vi "CALC_TRAN_TIME_SPAN_QUES.vi"(0 "VISA IN":refnum<visa-resource-name>, 5 "error in":errorcluster, 7 "Channel":i32) -> (11 "min":dbl, 13 "max":dbl, 14 "VISA Out":refnum<visa-resource-name>, 19 "error out":errorcluster)   [LabVIEW 2018, in "PNA-X.lvlib"]
doc: "CALCulate<cnum>:TRANsform:TIME:SPAN <num> \n1570\n\n(Read-Write) Sets the span time for time domain measurements. \nSee Critical Note \nParameters \n<cnum> Channel number of the measurement. There must be a selected measurement \non that channel. If unspecified, <cnum> is set to 1. \n<num> Span time in seconds; any number between: \n0 and 2* [(number of points-1) / frequency span] \nNote: This command will accept MIN or MAX instead of a numeric \nparameter. See SCPI Syntax for more information. \nExamples CALC:TRAN:TIME:SPAN 1e-8 \ncalculate2:transform:time:span maximum \nQuery Syntax CALCulate<cnum>:TRANsform:TIME:SPAN? \nReturn Type Numeric \nDefault 20 ns"
uses:
  PNA-X.lvlib
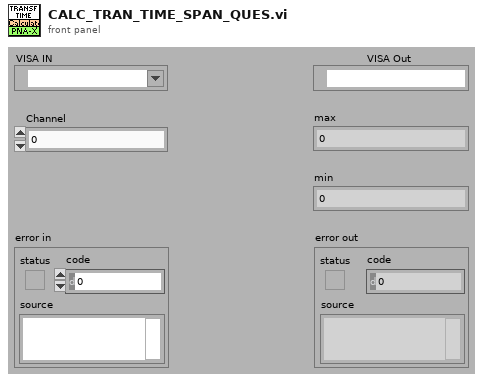
[diagram p1: front panel]
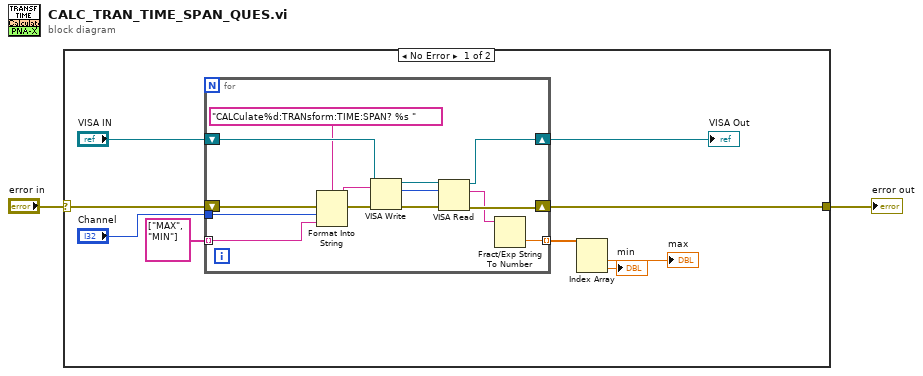
[diagram p0: block diagram]
diagram:
  n1 = case shown="No Error" "error in" {
    selector: "error in" -> [w11 w26]
    tunnel: [w9 w26] -> w1
    frame No Error {
      n2 = for {
        tunnel: "Channel" -> [w20]
        shift-right: [w15] -> w8
        shift-left: "VISA IN" -> [w22]
        shift-right: [w14] -> w9
        shift-left: w11 -> [w25]
        tunnel: string[] ["MAX", "MIN"] -> [w19] mode=indexing
        tunnel: [w12] -> w5 mode=indexing
        n3 = Format Into String(format string="CALCulate%d:TRANsform:TIME:SPAN? %s " ("Cmdline"), error in=w25, w20, w19) -> (resulting string=w23:string, error out=w24:errorcluster)  [unwired: 1 in]
        n4 = VISA Write(VISA resource name=w22, write buffer=w23, error in (no error)=w24) -> (VISA resource name out=w16:refnum<visa-resource-name>, return count=w17:u32, error out=w18:errorcluster)
        n5 = VISA Read(VISA resource name=w16, byte count=w17, error in (no error)=w18) -> (VISA resource name out=w15:refnum<visa-resource-name>, read buffer=w13:string, error out=w14:errorcluster)  [unwired: 1 out]
        n6 = Fract/Exp String To Number(string=w13) -> (number=w12:dbl)  [unwired: 3 in, 1 out]
      }
      "VISA Out" <- w8
      n7 = Index Array(array=w5) -> (element #1=→"max":dbl, element #2=→"min":dbl)  [unwired: 2 in]
    }
    frame Error {
    }
  }
  "error out" <- w1
